vi "Register Rotating Time File Sink as Default.vi"(8 "error in (no error)":errorcluster, 11 "Path":path) -> (0 "error out":errorcluster)   [LabVIEW 2020, in "LV Log.lvlib"]
uses:
  LV Log.lvlib
  Sinks/Rotating File Sink/Rotating Daily File Sink.lvclass
  C:/Users/hughe_cx/Documents/05_repos/LVLog/Source/Sinks/File Sink/File Sink.lvclass
  C:/Users/hughe_cx/Documents/05_repos/LVLog/Source/Sinks/Sink/Sink.lvclass
  C:/Users/hughe_cx/Documents/05_repos/LVLog/Source/Sinks/Rotating File Sink/Rotating Daily File Sink.lvclass
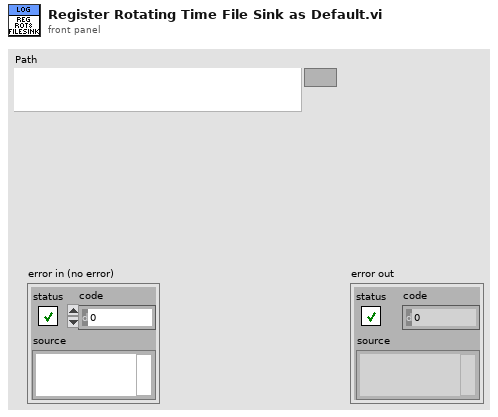
[diagram p1: front panel]
types:
  T1 = enum16{"Init", "Get Logger", "Register Sink", "Set Global Debug Level", "Get Sinks"}
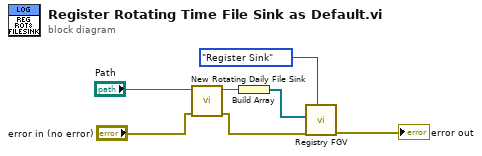
[diagram p0: block diagram]
diagram:
  n1 = call "New Rotating Daily File Sink.vi"("error in (no error)"="error in (no error)", "File Path"="Path") -> ("error out"=w3:errorcluster, "Rotating Daily File Sink out"=w1:refnum<class "Rotating Daily File Sink.lvclass">)  [unwired: 8 in]
  n2 = Build Array(w1) -> (w5:refnum<class "Rotating Daily File Sink.lvclass">[])
  n3 = call "Registry FGV.vi"("State (Get Logger)"=T1."Register Sink", "error in (no error)"=w3, "Sink(s)"=w5) -> ("error out"=→"error out":errorcluster)  [unwired: 5 in, 3 out]
